vi "Get Scaling Parameters.vi"   [LabVIEW 2020, in "SLSC.lvlib"]
doc: "Gets scaling parameters from a scale."
uses:
  <vilib>/SLSC/SLSC.lvlib
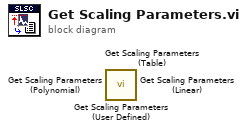
[diagram p0: block diagram]
diagram:
  n1 = call <vilib>:"Get Scaling Parameters (User Defined).vi"() -> ()  [unwired: 11 in, 5 out]
  n2 = call <vilib>:"Get Scaling Parameters (Table).vi"() -> ()  [unwired: 10 in, 6 out]
  n3 = call <vilib>:"Get Scaling Parameters (Polynomial).vi"() -> ()  [unwired: 11 in, 5 out]
  n4 = call <vilib>:"Get Scaling Parameters (Linear).vi"() -> ()  [unwired: 11 in, 5 out]
